vi "DSC_Create Net Var.vi"   [LabVIEW 2016, in "data.citadel.lvclass"]
uses:
  data.citadel.lvclass
  <vilib>/lvdsc/NI_DSC.lvlib
types:
  T1 = cluster{"enable? (F)":bool, "data type (deprecated)":enum32{"U32 Bit Field", "Boolean", "Double", "String"}, "log data? (F)":bool, "log alarms & events? (F)":bool, "value resolution (for Float variables only)":dbl, "value deadband (for Float variables only)":dbl, "string logging format (for String variables only)":u32}
  T2 = enum32{"u32BitField", "bool", "double", "string", "int8", "uint8", "int16", "uint16", "int32", "uint32", "int64", "uint64", "single", "double waveform", "int16 waveform", "array of boolean", "array of int8", "array of uint8", "array of int16", "array of uint16", "array of int32", "array of uint32", "array of int64", "array of uint64", "array of single", "array of double", "array of double waveform", "array of int16 waveform", "array of string", "variant", "timestamp", "fixed point", "custom"}
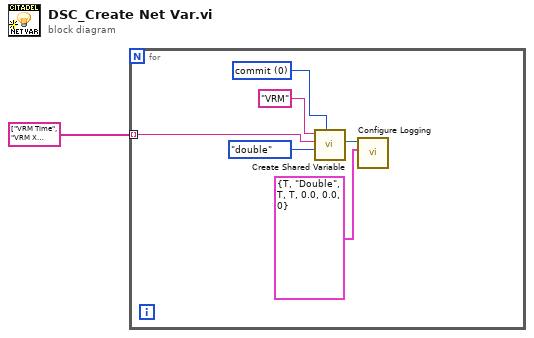
[diagram p0: block diagram]
diagram:
  n1 = for {
    tunnel: string[] ["VRM Time", "VRM X heaterPresent", "VRM Y heaterPresent", "VRM Z heaterPresent", "VRM X heater", "VRM Y heater", "VRM Z heater", "VRM X heater fault", "VRM Y heater fault", "VRM Z heater fault", "VRM X at rest", "VRM Y at rest", "VRM Z at rest", "VRM X setpT", "VRM Y setpT", "VRM Z setpT", "VRM X magT", "VRM Y magT", "VRM Z magT", "VRM X outT", "VRM Y outT", "VRM Z outT", "VRM X sweep", "VRM Y sweep", "VRM Z sweep", "VRM X magA", "VRM Y magA", "VRM Z magA", "VRM X outA", "VRM Y outA", "VRM Z outA", "VRM X meas A", "VRM Y meas A", "VRM Z meas A", "VRM X meas V", "VRM Y meas V", "VRM Z meas V", "VRM X sweep A", "VRM Y sweep A", "VRM Z sweep A", "VRM VrmX setpT", "VRM VrmY setpT", "VRM VrmZ setpT", "VRM VrmSweepMode", "VRM VrmSweepTime", "VRM VrmSweepRate", "VRM Vrm pers"] ("Array") -> [w2] mode=indexing
    w5 = u16 0 items=["commit", "buffer"] ("set mode")
    n2 = call <vilib>:"Create Shared Variable.vi"("set mode"=w5, "data type"=T2."double", "shared variable name"=w2, "process name"="VRM") -> ("shared variable"=w6:refnum<k21>)  [unwired: 5 in, 2 out]
    n3 = call <vilib>:"Configure Logging.vi"("logging settings"=T1 {"enable? (F)"=TRUE, "data type (deprecated)"=enum."Double", "log data? (F)"=TRUE, "log alarms & events? (F)"=TRUE, "value resolution (for Float variables only)"=0.0, "value deadband (for Float variables only)"=0.0, "string logging format (for String variables only)"=0}, "variable reference in"=w6) -> ()  [unwired: 8 in, 2 out]
  }
